vi "SPT-Init (Continuous).vi"(0 "Pulse Train Params":T2, 5 "Start Pulse Rate (Hz)":dbl, 7 "Start Phase (cycles)":dbl, 9 "Fs (Hz)":dbl, 11 "error in (no error)":errorcluster) -> (4 "Initial State":T1, 15 "error out":errorcluster)   [LabVIEW 2015]
uses:
  SPT-Properties.ctl
  SPT-Shape.ctl
  SPT-State.ctl
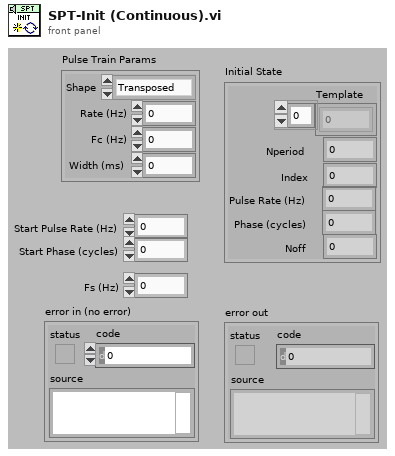
[diagram p1: front panel]
types:
  T1 = typedef "SPT-State.ctl" = cluster{"Template":dbl[], "Nperiod":i32, "Index":i32, "Pulse Rate (Hz)":dbl, "Phase (cycles)":dbl, "Noff":i32}
  T2 = typedef "SPT-Properties.ctl" = cluster{"Shape":T3, "Rate (Hz)":dbl, "Fc (Hz)":dbl, "Width (ms)":dbl}
  T3 = typedef "SPT-Shape.ctl" = enum16{"Transposed", "Alpha", "Gabor"}
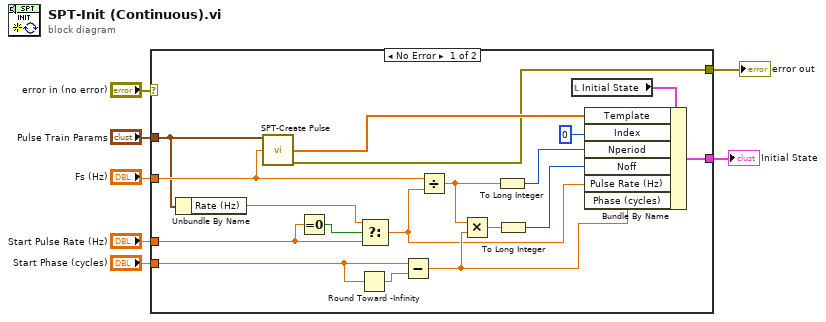
[diagram p0: block diagram]
diagram:
  n1 = case shown="No Error" "error in (no error)" {
    selector: "error in (no error)" -> [_ w26]
    tunnel: [w8 w26] -> w6
    tunnel: "Pulse Train Params" -> [w10 _]
    tunnel: "Fs (Hz)" -> [w12 _]
    tunnel: [w24 _] -> w3
    tunnel: "Start Pulse Rate (Hz)" -> [w14 _]
    tunnel: "Start Phase (cycles)" -> [w16 _]
    frame No Error {
      n2 = Unbundle By Name(w10) -> ("Rate (Hz)"=w9:dbl)
      n3 = call "SPT-Create Pulse.vi"("SPT.Properties"=w10, "Fs (Hz)"=w12) -> ("Pulse"=w11:dbl[], "error out"=w8:errorcluster)  [unwired: 12 in]
      n4 = Equal To 0?(x=w14) -> (x = 0?=w15:bool)
      n5 = Round Toward -Infinity(1:w16) -> (0:w17:dbl)
      n6 = Select(t=w9, s=w15, f=w14) -> (s? t:f=w13:dbl)
      n7 = Subtract(x=w16, y=w17) -> (x-y=w18:dbl)
      n8 = Divide(x=w12, y=w13) -> (x/y=w20:dbl)
      n9 = Multiply(x=w20, y=w18) -> (x*y=w23:dbl)
      n10 = To Long Integer(number=w20) -> (32bit integer=w19:i32)
      n11 = To Long Integer(number=w23) -> (32bit integer=w21:i32)
      n12 = local read "Initial State"() -> (w25:T1)
      n13 = Bundle By Name(cluster=w25, "Template"=w11, "Index"=0, "Nperiod"=w19, "Noff"=w21, "Pulse Rate (Hz)"=w13, "Phase (cycles)"=w18) -> (w24:T1)
    }
    frame Error {
    }
  }
  "error out" <- w6
  "Initial State" <- w3
